vi "Compressor Control.vi"() -> ()   [LabVIEW 2023]
doc: "This VI hosts two shared variables that can be accessed by a variety of client VIs. Shared Variables are typically used for monitoring lossy data, like memory usage, temperature data, etc."
uses:
  CM_Virtual_Panel_LV9_0.llb/Com_Set_AX.ctl
  <vilib>/Instr/_visa.llb/VISA Configure Serial Port (Serial Instr).vi
  <vilib>/Instr/_visa.llb/VISA Configure Serial Port (Instr).vi
panel:
  out "BPP Speed":dbl
  out "BPP status":bool
  out "SPP Speed":dbl
  out "SPP status":bool
  out "String 2":string="Hz"
  out "String":string="Hz"
  out "Unit 2":string="Torr"
  out "BPP Pressure":dbl=0.006515415732577395 format="%#_2e"
  out "Unit 4":string="Torr"
  out "overpressure indicator":bool
  out "Overpressure":bool
  out "Overpressure":bool
  out "output 1":dbl
  out "power":dbl(graph)
  out "Heater Power":string
  out "Cold head pressure":string
  out "Inlet pressure":dbl=1.198
  out "Monitor 1":cluster{"pressure":dbl, "Inlet pressure":dbl}(graph)
  in  "Reading 1":string(combo)="255:R:MRMD"
  out "Unit":string
  out "Unit":string="°C"
  out "Cold Head Temp":dbl=24.81
  out "Motor Current (A)":dbl(knob) scale=0.0..50.0
  out "Compressor Status":bool
  out "Overide status":bool
  out "Comp ON":bool
  out "?":cluster{dbl, dbl, dbl}(slide) scale=32.0..120.0
  out "?":cluster{dbl, dbl, dbl}(slide) scale=32.0..220.0
  out "?":cluster{dbl, dbl, dbl}(slide) scale=32.0..125.0
  out "?":cluster{dbl, dbl, dbl}(slide) scale=32.0..85.0
  out "DP":dbl(knob) scale=0.0..265.0
  in  "CM Tab Control":T1(tab)
  in  "COM PORT SETUP":T2={"Com Port #"=2, "Timeout(ms)"=500, "Baud"=115200, "Slave Address"=16, "LinkMode"=enum."SMDP-II:Checksum and stamp", "Num Retries"=0} {"Slave Address" min=16; "Com Port #" min=1}
  in  "Data Read Length":u32=20
  in  "Pressure Monitor Port":refnum<visa-resource-name>="COM5"
  in  "Command read length":u32=20
  in  "Separation length":i32=10
  in  "Do logging?":bool=TRUE
  in  "Log File Path":path
  out "error out":errorcluster
  out "data feedback":string
  out "command feedback":string
  in  "SPP Off/On":bool
  in  "SPP Standby/Full":bool
  in  "SPP port":refnum<visa-resource-name>
  in  "BPP Off/On":bool
  in  "BPP Standby/Full":bool
  in  "BPP port":refnum<visa-resource-name>
  in  "Set SPP standby speed":dbl=20.0 min=20.0 max=30.0 step=0.3000030517578125 format="%#.1f"
  in  "Set standby speed 3":bool
  out "SPP % full speed":i8 format="%.0f%%"
  in  "Set BPP standby speed":dbl=20.0 min=20.0 max=30.0 step=0.3000030517578125 format="%#.1f"
  out "BPP % full speed":i8 format="%.0f%%"
  out "SPP data out":bool
  out "BPP data out":bool
  in  "Set standby speed4":bool
  out "Gauge":cluster{dbl, dbl, dbl, dbl, dbl, dbl}(knob)={0.0, 0.0, -0.1, 0.0, 0.0, 0.0} scale=0.0..400.0
  in  "Additel 681 Tab Control":enum32{"Gauge Control", "Status"}(tab)
  in  "Zero Reading":bool
  in  "Cancel Zero reading":bool
  out "Gauge battery Voltage":dbl
  in  "Read":bool
  in  "Enable light control":bool
  in  "Gauge light":bool
  in  "Abort monitoring":bool
  out "Battery status":bool
  out "yellow":bool
  out "orange":bool
  out "red":bool
  in  "voltage read length":u32=25
  out "Voltage feedback":string
  in  "monitor 2 read length":u32=25
  out "monitor 2 feedback":string
  in  "monitor 1 read length":u32=25
  out "Monitor 1 feedback":string
  out "Unit":string="°C"
  out "Vapor Temp":dbl=24.81
  out "Monitor 2":dbl(graph)=24.81
  in  "Reading 2":string(combo)="255:R:OTEMP"
  out "Monitor 3":dbl(graph)=0.006479277826451128
  out "SPP Pressure":dbl=0.006479277826451128 format="%#_2e"
  out "Monitor 4":T3(graph)
  in  "Compressor Relay Control":enum32{"Normal", "Overide"}(tab)
  in  "Pressure Upper Limit":dbl=3.0
  out "Helium Overpressure":bool
  in  "Pressure Lower Limit":dbl=1.0
  in  "Set Relay voltage":dbl(slide)=9.0 scale=0.0..10.0
  out "Numeric 2":dbl=9.0
  out "Helium underpressure":bool
  in  "Compressor On":bool caption="Compressor Ona"
  # "Additel Pressure Gauge"
  # "Cryomech Liquefier"
  # "Pressure (Psi)"
  # "Cryomech Control"
  # "Min"
  # "Max"
  # "Latest"
  # "Coolant Supply"
  # "Coolant Return"
  # "Exchage Helium"
  # "Motor Oil"
  # "Temperature °F"
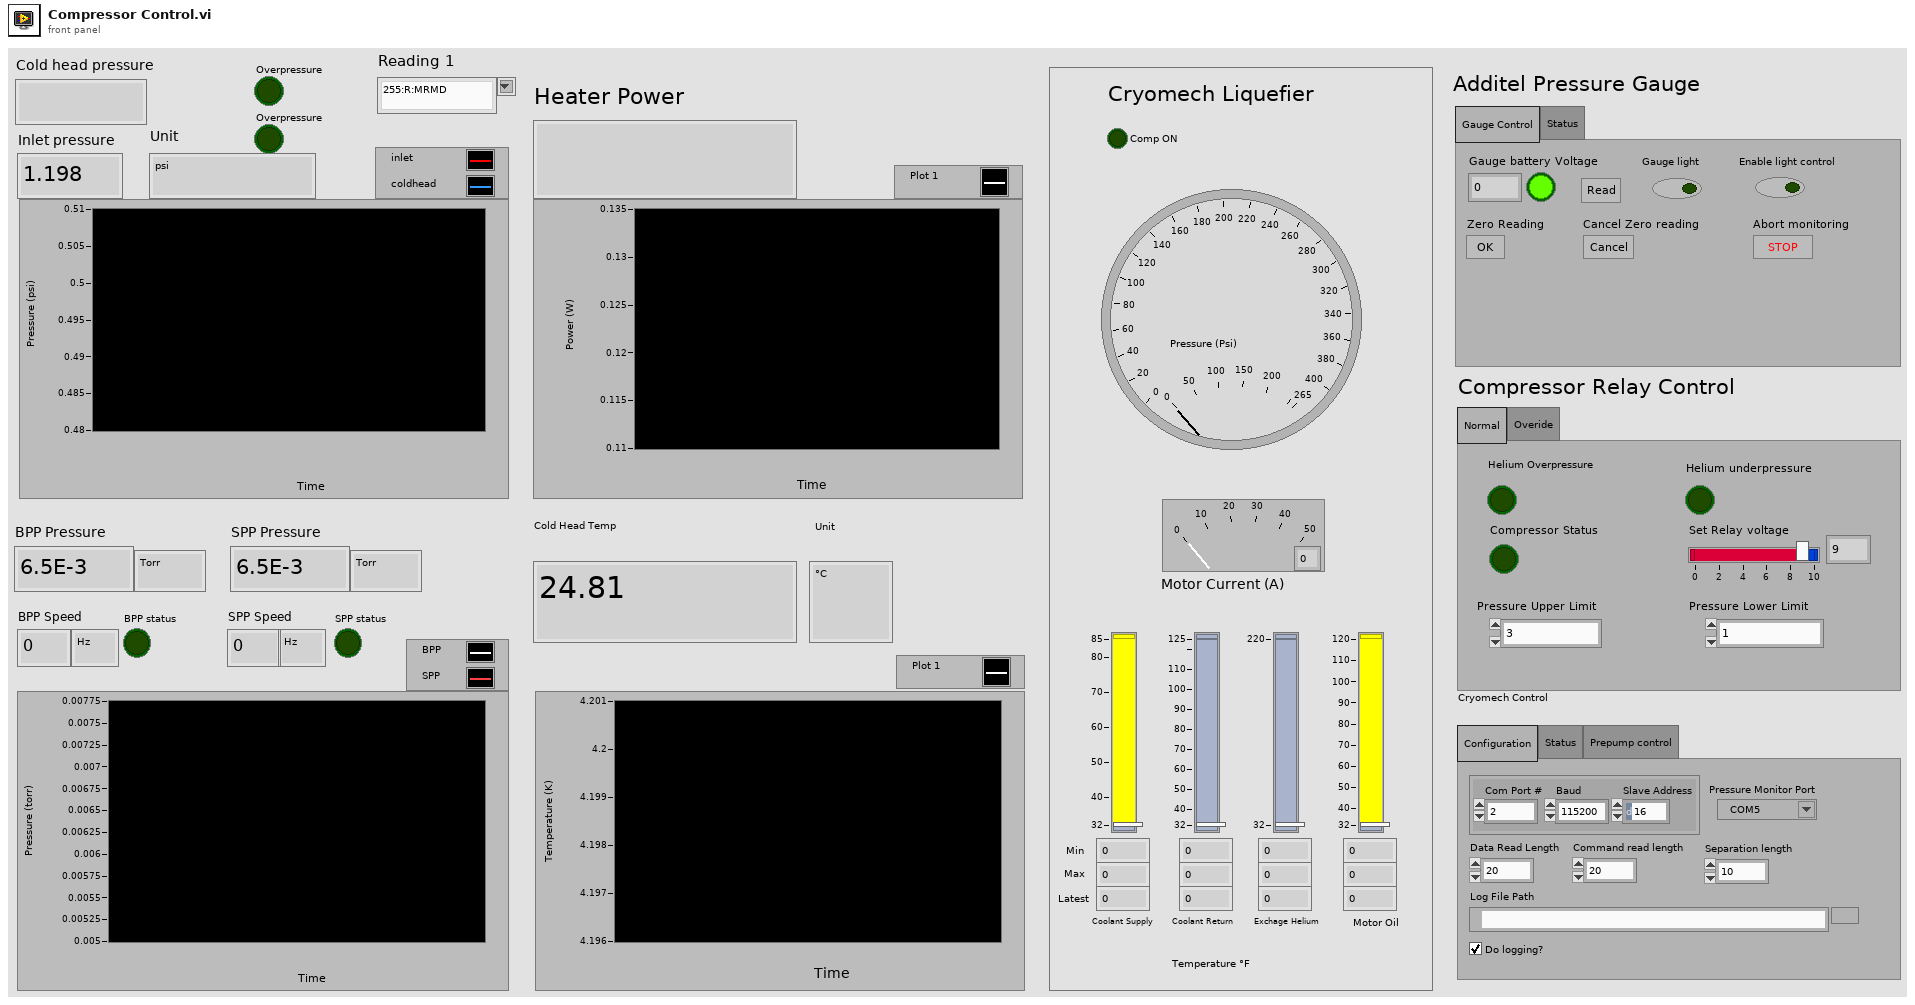
[diagram p1: front panel]
types:
  T1 = enum32{"Configuration", "Status", "Prepump control"}
  T2 = typedef "Com_Set_AX.ctl" = cluster{"Com Port #":u8, "Timeout(ms)":u32, "Baud":u32, "Slave Address":u8, "LinkMode":enum16{"SMDP-I:Checksum, no stamp", "SMDP-II:Checksum and stamp", "Sycon Protocol"}, "Num Retries":u8}
  T3 = cluster{"Output Variable 1":dbl, "Output Variable 2":dbl}
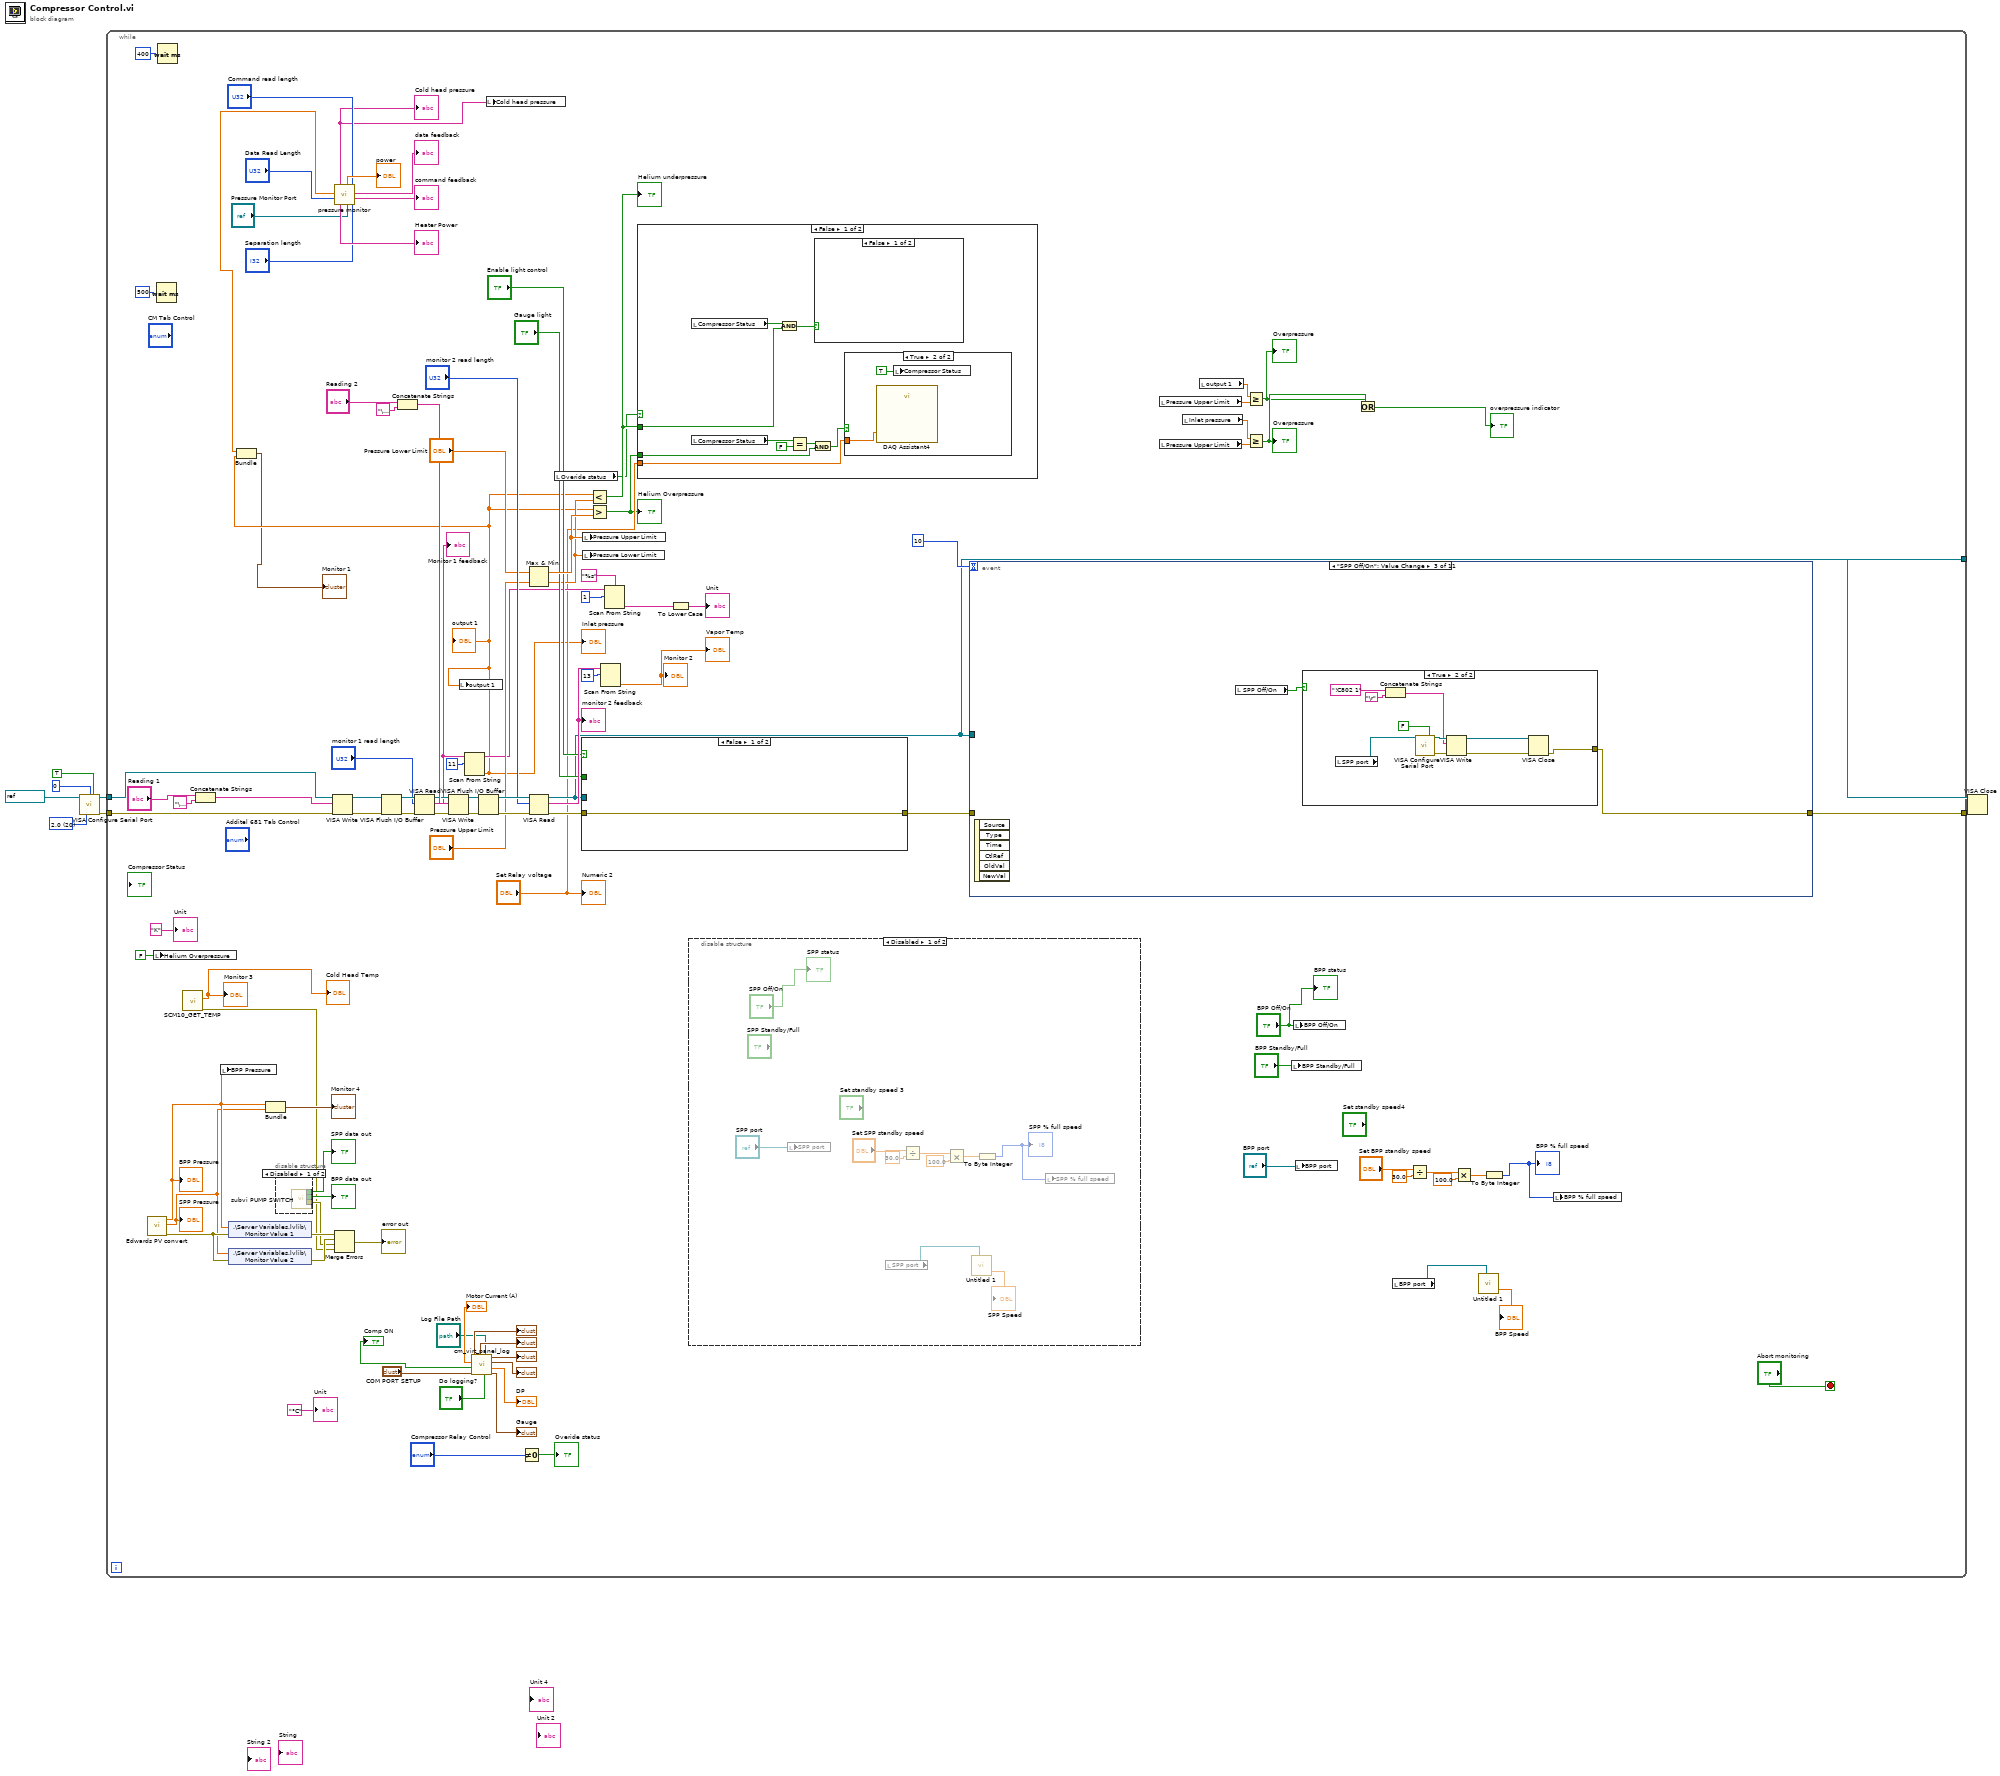
[diagram p0: block diagram]
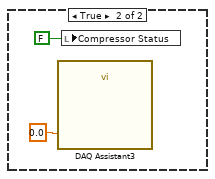
[diagram p4: hidden frame]
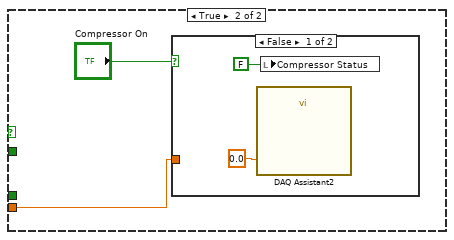
[diagram p6: hidden frame]
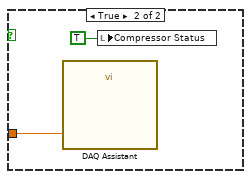
[diagram p7: hidden frame]
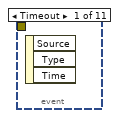
[diagram p8: hidden frame]
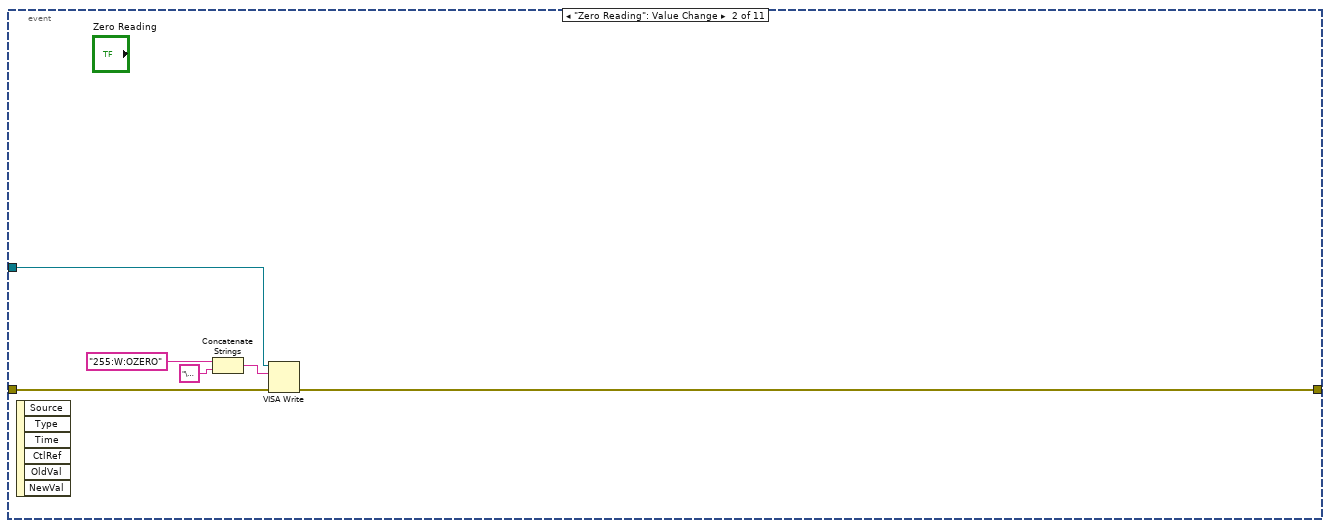
[diagram p9: hidden frame]
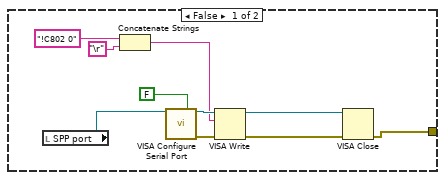
[diagram p10: hidden frame]
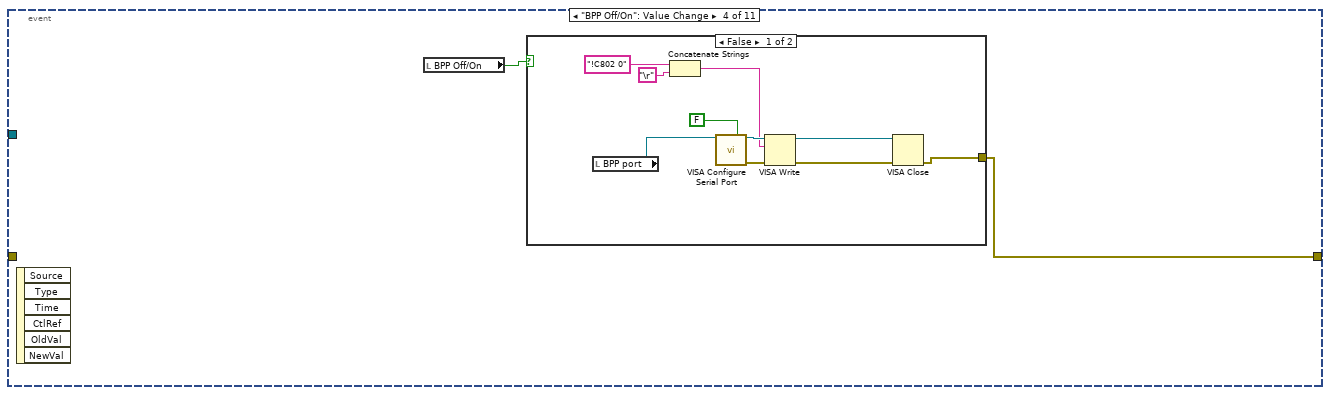
[diagram p11: hidden frame]
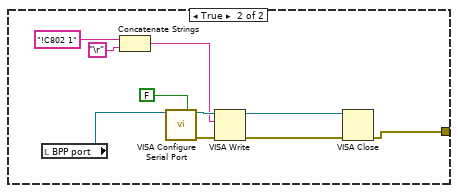
[diagram p12: hidden frame]
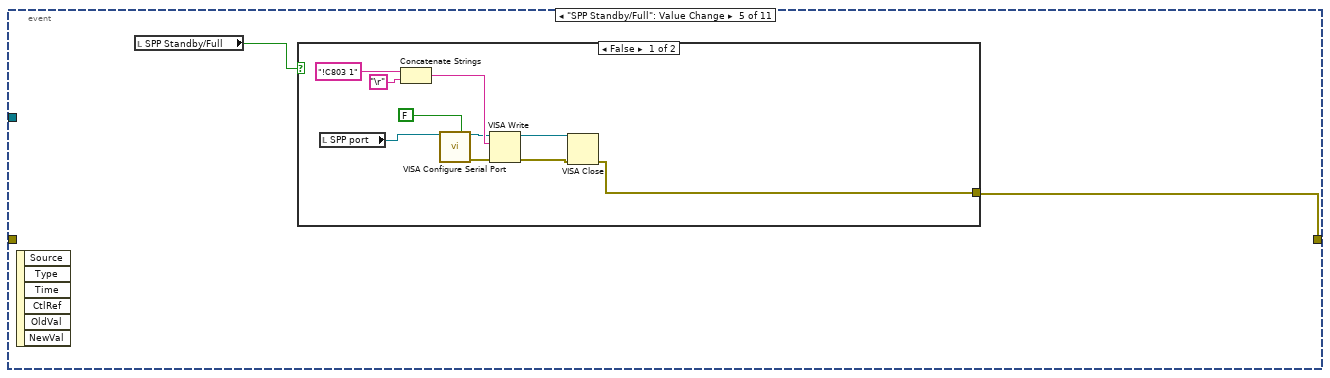
[diagram p13: hidden frame]
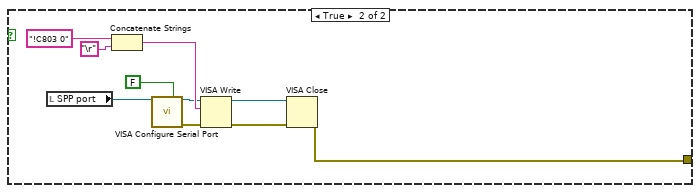
[diagram p14: hidden frame]
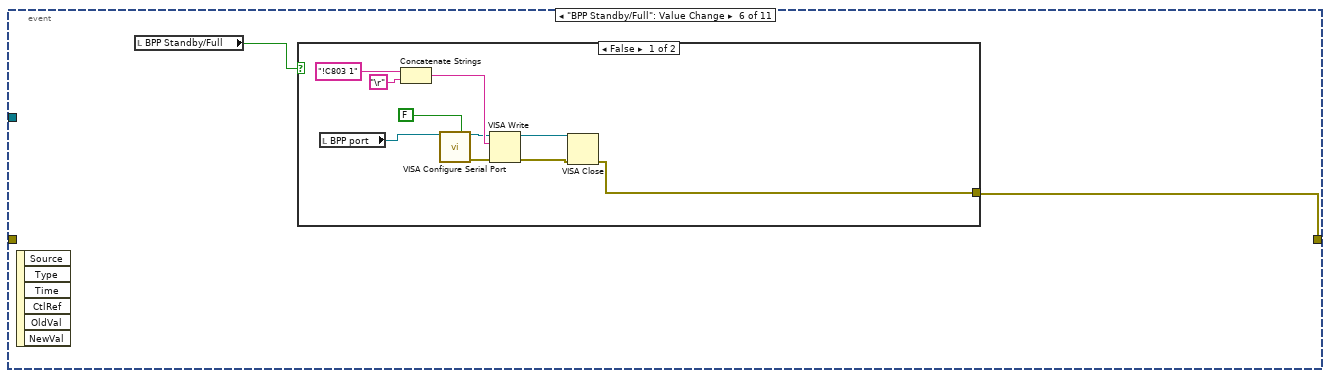
[diagram p15: hidden frame]
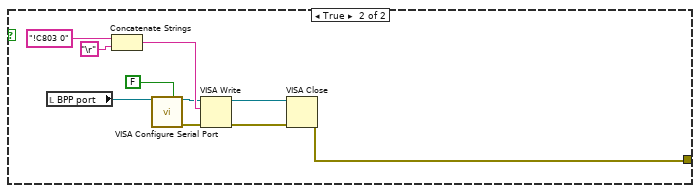
[diagram p16: hidden frame]
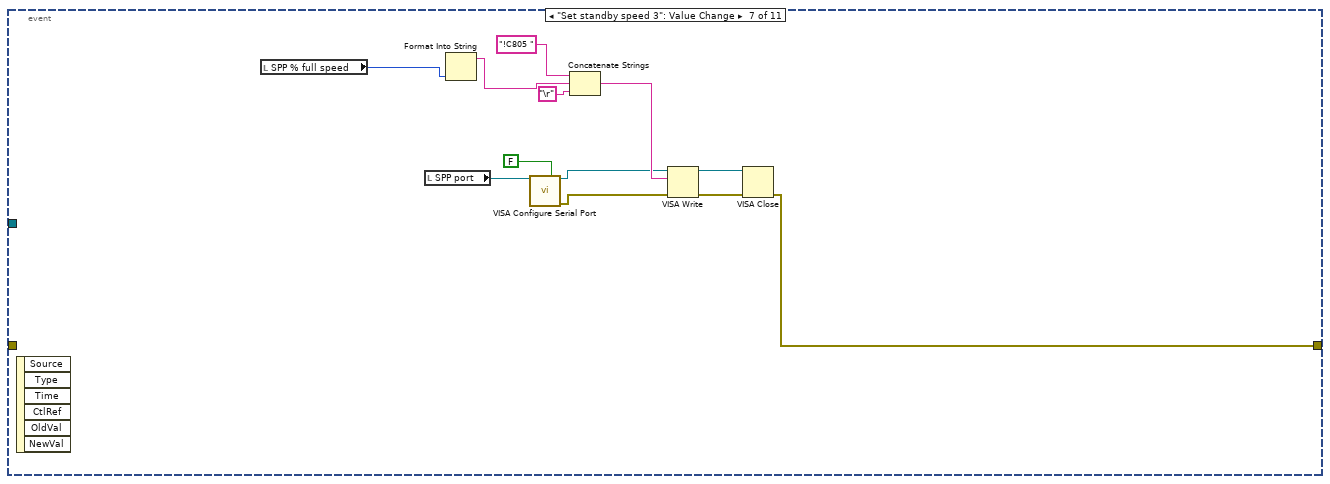
[diagram p17: hidden frame]
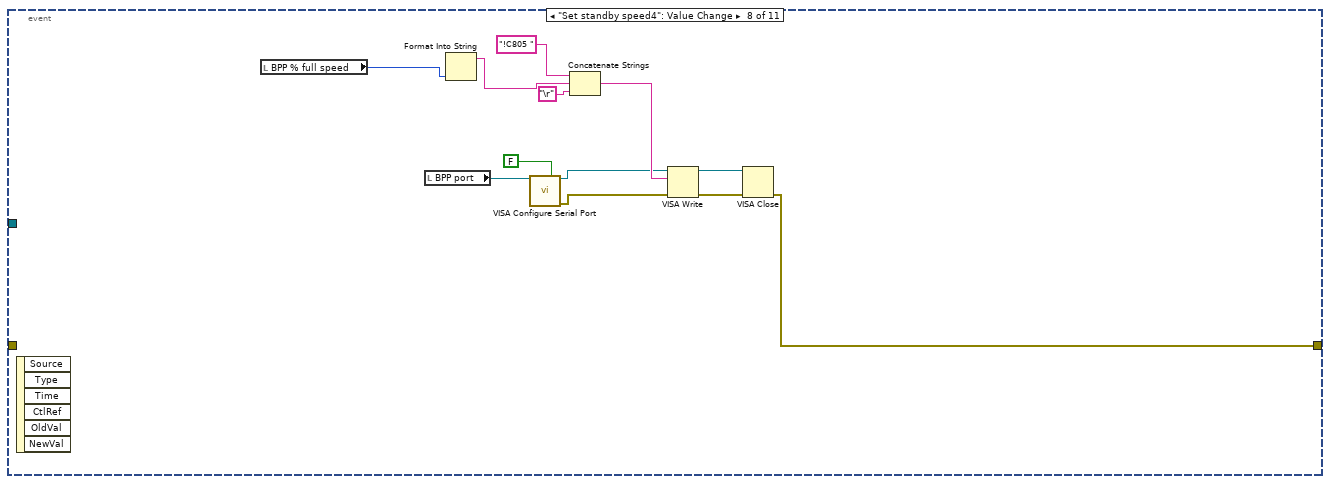
[diagram p18: hidden frame]
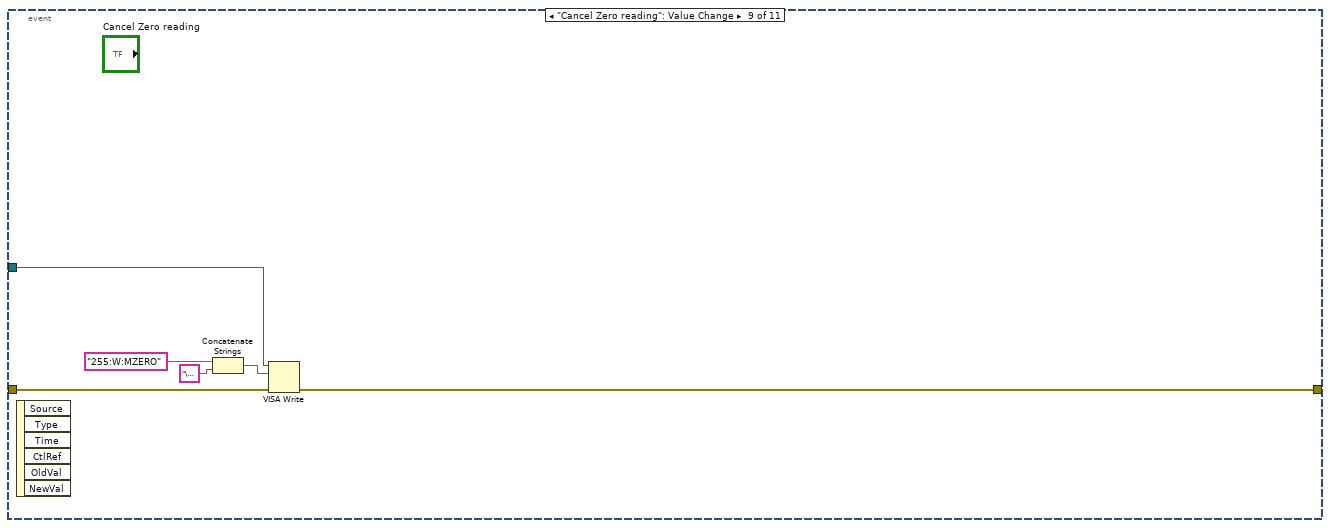
[diagram p19: hidden frame]
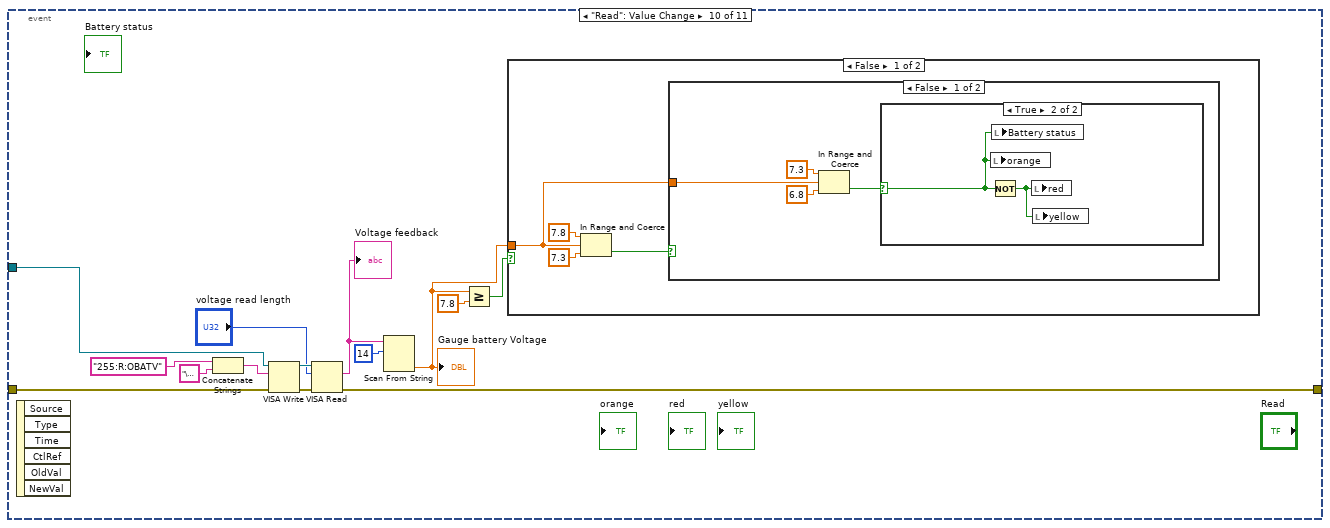
[diagram p20: hidden frame]
diagram:
  w5 = u16 20 items=["1.0"=10, "1.5"=15, "2.0"=20] ("stop bits (10: 1 bit)")
  n1 = call-poly "VISA Configure Serial Port"("VISA resource name"=refnum<visa-resource-name> "COM3", "termination char\n(0xA = '\\n' = LF)"=u8 0 ("termination char\n(0xA = '\\n' = LF)"), "Enable Termination\nChar (T)"=TRUE ("Enable Termination\nChar (T)"), "stop bits (10: 1 bit)"=w5) -> ("VISA resource name out"=w3:refnum<visa-resource-name>, "error out"=w4:errorcluster)  [unwired: 10 in]
  n2 = while {
    tunnel: [w82] -> w2
    tunnel: w4 -> [w61]
    tunnel: w3 -> [w88]
    tunnel: [w81] -> w1
    stop <- "Abort monitoring" stop-if-true
    n3 = call "Edwards PV convert.vi"() -> ("error out"=w64:errorcluster, "Output Variable 2"=w54:dbl, "Output Variable 1"=w55:dbl)  [unwired: 9 in]
    "SPP Pressure" <- w54
    "BPP Pressure" <- w55
    n4 = local write "Helium Overpressure"(FALSE ("Helium Overpressure")) -> ()
    n5 = Wait (ms)(milliseconds to wait=u32 500) -> ()  [unwired: 1 out]
    n6 = Wait (ms)(milliseconds to wait=u32 400) -> ()  [unwired: 1 out]
    n7 = call "SCM10_GET_TEMP.vi"() -> ("ERR OUT"=w52:errorcluster, "Temperature (K)"=→"Monitor 3" →"Cold Head Temp":dbl)  [unwired: 9 in, 1 out]
    n8 = Concatenate Strings("Reading 1", "\u0000") -> (w114:string)
    n9 = local write "BPP Pressure"(w55) -> ()
    n10 = shared-variable ".\\Server Variables.lvlib\\Monitor Value 1"(w55, error in=w64) -> (error out=w63:errorcluster)
    n11 = shared-variable ".\\Server Variables.lvlib\\Monitor Value 2"(w54, error in=w64) -> (error out=w62:errorcluster)
    n12 = Bundle("Output Variable 1"=w55, "Output Variable 2"=w54) -> (→"Monitor 4":T3)  [unwired: 1 in]
    n13 = disable-structure shown="Disabled" {
      disable-tunnel: [w117 _] -> w69
      disable-tunnel: [w116 _] -> w68
      disable-tunnel: [w115 _] -> w60
      frame Disabled {
        n14 = call "subvi PUMP SWITCH.vi"() -> ("error out"=w115:errorcluster, "data out"=w117:bool, "data out 2"=w116:bool)  [unwired: 9 in]
      }
      frame Enabled {
      }
    }
    "BPP data out" <- w69
    "SPP data out" <- w68
    n15 = VISA Write(VISA resource name=w88, write buffer=w114, error in (no error)=w61) -> (VISA resource name out=w110:refnum<visa-resource-name>, error out=w112:errorcluster)  [unwired: 1 out]
    n16 = call "pressure monitor.vi"("Data Read Length"="Data Read Length", "Pressure Monitor Port"="Pressure Monitor Port", "Command read length"="Command read length", "Separation length"="Separation length") -> ("Cold head pressure"=w24:string, "pressure"=w23:dbl, "Heater Power"=→"Heater Power":string, "power"=→"power":dbl, "data feedback"=→"data feedback":string, "command feedback"=→"command feedback":string)
    "Cold head pressure" <- w24
    n17 = Merge Errors(w63, w62, w60, w52) -> (→"error out":errorcluster)
    n18 = VISA Flush I/O Buffer(VISA resource name=w110, error in (no error)=w112) -> (VISA resource name out=w111:refnum<visa-resource-name>, error out=w107:errorcluster)  [unwired: 1 in]
    n19 = Concatenate Strings("Reading 2", "\u0000") -> (w103:string)
    n20 = VISA Read(VISA resource name=w111, byte count="monitor 1 read length", error in (no error)=w107) -> (VISA resource name out=w93:refnum<visa-resource-name>, read buffer=w79:string, error out=w92:errorcluster)  [unwired: 1 out]
    "Monitor 1 feedback" <- w79
    n21 = VISA Write(VISA resource name=w93, write buffer=w103, error in (no error)=w92) -> (VISA resource name out=w99:refnum<visa-resource-name>, error out=w101:errorcluster)  [unwired: 1 out]
    n22 = Scan From String(input string=w79, initial scan location=u32 11) -> (remaining string=w77:string, output 1=w22:dbl)  [unwired: 3 in, 2 out]
    "Inlet pressure" <- w22
    "output 1" <- w22
    n23 = Bundle("pressure"=w23, "Inlet pressure"=w22) -> (→"Monitor 1":cluster{"pressure":dbl, "Inlet pressure":dbl})  [unwired: 1 in]
    n24 = local write "output 1"(w22) -> ()
    n25 = call "cm_virt_panel_log.vi"("Do logging?"="Do logging?", "Log File Path"="Log File Path", "COM PORT SETUP"="COM PORT SETUP") -> ("Gauge"=→"Gauge":cluster{dbl, dbl, dbl, dbl, dbl, dbl}, "DP"=→"DP":dbl, "H2O IN"=→"?":cluster{dbl, dbl, dbl}, "H2O OUT"=→"?":cluster{dbl, dbl, dbl}, "He GAS"=→"?":cluster{dbl, dbl, dbl}, "Comp ON"=→"Comp ON":bool, "Motor Amps"=→"Motor Current (A)":dbl, "OIL TEMP"=→"?":cluster{dbl, dbl, dbl})  [unwired: 1 in]
    n26 = VISA Flush I/O Buffer(VISA resource name=w99, error in (no error)=w101) -> (VISA resource name out=w100:refnum<visa-resource-name>, error out=w95:errorcluster)  [unwired: 1 in]
    n27 = local write "Cold head pressure"(w24) -> ()
    n28 = Not Equal To 0?(x="Compressor Relay Control") -> (x != 0?=→"Overide status":bool)
    n29 = Max & Min(x="Pressure Lower Limit", y="Pressure Upper Limit") -> (max(x,y)=w89:dbl, min(x,y)=w73:dbl)
    n30 = VISA Read(VISA resource name=w100, byte count="monitor 2 read length", error in (no error)=w95) -> (VISA resource name out=w82:refnum<visa-resource-name>, read buffer=w97:string, error out=w85:errorcluster)  [unwired: 1 out]
    "monitor 2 feedback" <- w97
    n31 = local read "Overide status"() -> (w58:bool)
    n32 = case shown="False" "Enable light control" {
      tunnel: "Gauge light" -> [_ w319]
      tunnel: w85 -> [w315 w318]
      tunnel: [w315 w317] -> w80
      tunnel: w82 -> [_ w316]
      frame False {
      }
      frame True {
        n33 = case shown="False" w319 {
          tunnel: w316 -> [w322 w331]
          tunnel: [w321 w327] -> w317
          tunnel: w318 -> [w320 w326]
          frame False {
            n34 = Concatenate Strings("255:W:OBLAC:0" ("string"), "\u0000" ("string")) -> (w323:string)
            n35 = VISA Write(VISA resource name=w322, write buffer=w323, error in (no error)=w320) -> (error out=w321:errorcluster)  [unwired: 2 out]
          }
          frame True {
            n36 = Concatenate Strings("255:W:OBLAC:1" ("string"), "\u0000" ("string")) -> (w328:string)
            n37 = VISA Write(VISA resource name=w331, write buffer=w328, error in (no error)=w326) -> (error out=w327:errorcluster)  [unwired: 2 out]
          }
        }
      }
    }
    n38 = local write "Pressure Upper Limit"(w89) -> ()
    n39 = local write "Pressure Lower Limit"(w73) -> ()
    n40 = Less?(x=w22, y=w73) -> (x < y?=w65:bool)
    "Helium underpressure" <- w65
    n41 = Greater?(x=w22, y=w89) -> (0:w66:bool)
    "Helium Overpressure" <- w66
    n42 = Scan From String(input string=w97, initial scan location=u32 13) -> (output 1=→"Vapor Temp" →"Monitor 2":dbl)  [unwired: 3 in, 3 out]
    n43 = Scan From String(format string="%s", input string=w77, initial scan location=u32 1) -> (output 1=w75:string)  [unwired: 2 in, 3 out]
    n44 = case shown="False" w58 {
      tunnel: "Set Relay voltage" -> [w133 w141]
      tunnel: w66 -> [w129 _]
      tunnel: w65 -> [w128 _]
      frame False {
        n45 = local read "Compressor Status"() -> (w136:bool)
        n46 = local read "Compressor Status"() -> (w132:bool)
        n47 = And(x=w136, y=w128) -> (x .and. y?=w135:bool)
        n48 = Equal?(x=w132, y=FALSE) -> (x = y?=w130:bool)
        n49 = And(x=w130, y=w129) -> (x .and. y?=w134:bool)
        n50 = case shown="False" w135 {
          frame False {
          }
          frame True {
            n51 = call "DAQ Assistant3"("data"=0.0) -> ()  [unwired: 17 in, 2 out]
            n52 = local write "Compressor Status"(FALSE ("Compressor Status")) -> ()
          }
        }
        n53 = case shown="True" w134 {
          tunnel: w133 -> [_ w140]
          frame False {
          }
          frame True {
            n54 = call "DAQ Assistant4"("data"=w140) -> ()  [unwired: 17 in, 2 out]
            n55 = local write "Compressor Status"(TRUE ("Compressor Status")) -> ()
          }
        }
      }
      frame True {
        n56 = case shown="False" "Compressor On" {
          tunnel: w141 -> [_ w146]
          frame False {
            n57 = call "DAQ Assistant2"("data"=0.0) -> ()  [unwired: 17 in, 2 out]
            n58 = local write "Compressor Status"(FALSE ("Compressor Status")) -> ()
          }
          frame True {
            n59 = call "DAQ Assistant"("data"=w146) -> ()  [unwired: 17 in, 2 out]
            n60 = local write "Compressor Status"(TRUE ("Compressor Status")) -> ()
          }
        }
      }
    }
    n61 = To Lower Case(string=w75) -> (all lower case string=→"Unit":string)
    n62 = disable-structure shown="Disabled" {
      frame Disabled {
        n63 = local write "SPP port"("SPP port") -> ()
        n64 = local read "SPP port"() -> (w118:refnum<visa-resource-name>)
        n65 = Divide(x="Set SPP standby speed", y=30.0) -> (x/y=w124:dbl)
        n66 = Multiply(x=w124, y=sgl 100.0) -> (x*y=w127:dbl)
        n67 = call "Untitled 1.vi"("VISA resource name"=w118) -> ("Speed"=→"SPP Speed":dbl)  [unwired: 10 in]
        n68 = To Byte Integer(number=w127) -> (8bit integer=w120:i8)
        "SPP % full speed" <- w120
        n69 = local write "SPP % full speed"(w120) -> ()
        "SPP status" <- "SPP Off/On"
      }
      frame Enabled {
      }
    }
    n70 = event shown="[2] \"SPP Off/On\": Value Change" {
      selector: _ -> [_ _ _ _ _ _ _ _ _ _ _]
      dyn-events: _ -> [_ _ _ _ _ _ _ _ _ _ _]
      timeout: 10 -> [_ _ _ _ _ _ _ _ _ _ _]
      tunnel: w82 -> [_ w147 _ _ _ _ _ _ w266 w276 _]
      tunnel: [_ w148 w153 w175 w197 w219 w241 w253 w265 w275 _] -> w81
      tunnel: w80 -> [_ w149 _ _ _ _ _ _ w267 w272 _]
      event Timeout {
        n71 = event-data() -> ()  [unwired: 1 in, 3 out]
      }
      event "Zero Reading": Value Change {
        n72 = event-data() -> ()  [unwired: 1 in, 6 out]
        n73 = Concatenate Strings("255:W:OZERO" ("string"), "\u0000" ("string")) -> (w150:string)
        n74 = VISA Write(VISA resource name=w147, write buffer=w150, error in (no error)=w149) -> (error out=w148:errorcluster)  [unwired: 2 out]
      }
      event "SPP Off/On": Value Change {
        n75 = event-data() -> ()  [unwired: 1 in, 6 out]
        n76 = local read "SPP Off/On"() -> (w154:bool)
        n77 = case shown="True" w154 {
          tunnel: [w158 w168] -> w153
          frame False {
            n78 = local read "SPP port"() -> (w157:refnum<visa-resource-name>)
            n79 = Concatenate Strings("!C802 0" ("string"), "\r" ("string")) -> (w159:string)
            n80 = call-poly "VISA Configure Serial Port"("VISA resource name"=w157, "Enable Termination\nChar (T)"=FALSE ("Enable Termination\nChar (T)")) -> ("VISA resource name out"=w164:refnum<visa-resource-name>, "error out"=w163:errorcluster)  [unwired: 12 in]
            n81 = VISA Write(VISA resource name=w164, write buffer=w159, error in (no error)=w163) -> (VISA resource name out=w156:refnum<visa-resource-name>, error out=w155:errorcluster)  [unwired: 1 out]
            n82 = VISA Close(VISA resource name=w156, error in (no error)=w155) -> (error out=w158:errorcluster)
          }
          frame True {
            n83 = local read "SPP port"() -> (w167:refnum<visa-resource-name>)
            n84 = Concatenate Strings("!C802 1" ("string"), "\r" ("string")) -> (w169:string)
            n85 = call-poly "VISA Configure Serial Port"("VISA resource name"=w167, "Enable Termination\nChar (T)"=FALSE ("Enable Termination\nChar (T)")) -> ("VISA resource name out"=w174:refnum<visa-resource-name>, "error out"=w173:errorcluster)  [unwired: 12 in]
            n86 = VISA Write(VISA resource name=w174, write buffer=w169, error in (no error)=w173) -> (VISA resource name out=w166:refnum<visa-resource-name>, error out=w165:errorcluster)  [unwired: 1 out]
            n87 = VISA Close(VISA resource name=w166, error in (no error)=w165) -> (error out=w168:errorcluster)
          }
        }
      }
      event "BPP Off/On": Value Change {
        n88 = event-data() -> ()  [unwired: 1 in, 6 out]
        n89 = local read "BPP Off/On"() -> (w176:bool)
        n90 = case shown="False" w176 {
          tunnel: [w180 w190] -> w175
          frame False {
            n91 = local read "BPP port"() -> (w179:refnum<visa-resource-name>)
            n92 = Concatenate Strings("!C802 0" ("string"), "\r" ("string")) -> (w181:string)
            n93 = call-poly "VISA Configure Serial Port"("VISA resource name"=w179, "Enable Termination\nChar (T)"=FALSE ("Enable Termination\nChar (T)")) -> ("VISA resource name out"=w186:refnum<visa-resource-name>, "error out"=w185:errorcluster)  [unwired: 12 in]
            n94 = VISA Write(VISA resource name=w186, write buffer=w181, error in (no error)=w185) -> (VISA resource name out=w178:refnum<visa-resource-name>, error out=w177:errorcluster)  [unwired: 1 out]
            n95 = VISA Close(VISA resource name=w178, error in (no error)=w177) -> (error out=w180:errorcluster)
          }
          frame True {
            n96 = local read "BPP port"() -> (w189:refnum<visa-resource-name>)
            n97 = Concatenate Strings("!C802 1" ("string"), "\r" ("string")) -> (w191:string)
            n98 = call-poly "VISA Configure Serial Port"("VISA resource name"=w189, "Enable Termination\nChar (T)"=FALSE ("Enable Termination\nChar (T)")) -> ("VISA resource name out"=w196:refnum<visa-resource-name>, "error out"=w195:errorcluster)  [unwired: 12 in]
            n99 = VISA Write(VISA resource name=w196, write buffer=w191, error in (no error)=w195) -> (VISA resource name out=w188:refnum<visa-resource-name>, error out=w187:errorcluster)  [unwired: 1 out]
            n100 = VISA Close(VISA resource name=w188, error in (no error)=w187) -> (error out=w190:errorcluster)
          }
        }
      }
      event "SPP Standby/Full": Value Change {
        n101 = event-data() -> ()  [unwired: 1 in, 6 out]
        n102 = local read "SPP Standby/Full"() -> (w198:bool)
        n103 = case shown="False" w198 {
          tunnel: [w199 w209] -> w197
          frame False {
            n104 = local read "SPP port"() -> (w204:refnum<visa-resource-name>)
            n105 = Concatenate Strings("!C803 1" ("string"), "\r") -> (w208:string)
            n106 = call-poly "VISA Configure Serial Port"("VISA resource name"=w204, "Enable Termination\nChar (T)"=FALSE ("Enable Termination\nChar (T)")) -> ("VISA resource name out"=w203:refnum<visa-resource-name>, "error out"=w202:errorcluster)  [unwired: 12 in]
            n107 = VISA Write(VISA resource name=w203, write buffer=w208, error in (no error)=w202) -> (VISA resource name out=w201:refnum<visa-resource-name>, error out=w200:errorcluster)  [unwired: 1 out]
            n108 = VISA Close(VISA resource name=w201, error in (no error)=w200) -> (error out=w199:errorcluster)
          }
          frame True {
            n109 = local read "SPP port"() -> (w215:refnum<visa-resource-name>)
            n110 = Concatenate Strings("!C803 0" ("string"), "\r") -> (w218:string)
            n111 = call-poly "VISA Configure Serial Port"("VISA resource name"=w215, "Enable Termination\nChar (T)"=FALSE ("Enable Termination\nChar (T)")) -> ("VISA resource name out"=w213:refnum<visa-resource-name>, "error out"=w212:errorcluster)  [unwired: 12 in]
            n112 = VISA Write(VISA resource name=w213, write buffer=w218, error in (no error)=w212) -> (VISA resource name out=w211:refnum<visa-resource-name>, error out=w210:errorcluster)  [unwired: 1 out]
            n113 = VISA Close(VISA resource name=w211, error in (no error)=w210) -> (error out=w209:errorcluster)
          }
        }
      }
      event "BPP Standby/Full": Value Change {
        n114 = event-data() -> ()  [unwired: 1 in, 6 out]
        n115 = local read "BPP Standby/Full"() -> (w220:bool)
        n116 = case shown="False" w220 {
          tunnel: [w221 w231] -> w219
          frame False {
            n117 = local read "BPP port"() -> (w226:refnum<visa-resource-name>)
            n118 = Concatenate Strings("!C803 1" ("string"), "\r") -> (w230:string)
            n119 = call-poly "VISA Configure Serial Port"("VISA resource name"=w226, "Enable Termination\nChar (T)"=FALSE ("Enable Termination\nChar (T)")) -> ("VISA resource name out"=w225:refnum<visa-resource-name>, "error out"=w224:errorcluster)  [unwired: 12 in]
            n120 = VISA Write(VISA resource name=w225, write buffer=w230, error in (no error)=w224) -> (VISA resource name out=w223:refnum<visa-resource-name>, error out=w222:errorcluster)  [unwired: 1 out]
            n121 = VISA Close(VISA resource name=w223, error in (no error)=w222) -> (error out=w221:errorcluster)
          }
          frame True {
            n122 = local read "BPP port"() -> (w237:refnum<visa-resource-name>)
            n123 = Concatenate Strings("!C803 0" ("string"), "\r") -> (w240:string)
            n124 = call-poly "VISA Configure Serial Port"("VISA resource name"=w237, "Enable Termination\nChar (T)"=FALSE ("Enable Termination\nChar (T)")) -> ("VISA resource name out"=w235:refnum<visa-resource-name>, "error out"=w234:errorcluster)  [unwired: 12 in]
            n125 = VISA Write(VISA resource name=w235, write buffer=w240, error in (no error)=w234) -> (VISA resource name out=w233:refnum<visa-resource-name>, error out=w232:errorcluster)  [unwired: 1 out]
            n126 = VISA Close(VISA resource name=w233, error in (no error)=w232) -> (error out=w231:errorcluster)
          }
        }
      }
      event "Set standby speed 3": Value Change {
        n127 = event-data() -> ()  [unwired: 1 in, 6 out]
        n128 = local read "SPP % full speed"() -> (w248:i8)
        n129 = local read "SPP port"() -> (w246:refnum<visa-resource-name>)
        n130 = Format Into String(w248) -> (resulting string=w250:string)  [unwired: 3 in, 1 out]
        n131 = call-poly "VISA Configure Serial Port"("VISA resource name"=w246, "Enable Termination\nChar (T)"=FALSE ("Enable Termination\nChar (T)")) -> ("VISA resource name out"=w245:refnum<visa-resource-name>, "error out"=w244:errorcluster)  [unwired: 12 in]
        n132 = Concatenate Strings("!C805 " ("string"), w250, "\r" ("string")) -> (w252:string)
        n133 = VISA Write(VISA resource name=w245, write buffer=w252, error in (no error)=w244) -> (VISA resource name out=w243:refnum<visa-resource-name>, error out=w242:errorcluster)  [unwired: 1 out]
        n134 = VISA Close(VISA resource name=w243, error in (no error)=w242) -> (error out=w241:errorcluster)
      }
      event "Set standby speed4": Value Change {
        n135 = event-data() -> ()  [unwired: 1 in, 6 out]
        n136 = local read "BPP % full speed"() -> (w260:i8)
        n137 = local read "BPP port"() -> (w258:refnum<visa-resource-name>)
        n138 = Format Into String(w260) -> (resulting string=w262:string)  [unwired: 3 in, 1 out]
        n139 = call-poly "VISA Configure Serial Port"("VISA resource name"=w258, "Enable Termination\nChar (T)"=FALSE ("Enable Termination\nChar (T)")) -> ("VISA resource name out"=w257:refnum<visa-resource-name>, "error out"=w256:errorcluster)  [unwired: 12 in]
        n140 = Concatenate Strings("!C805 " ("string"), w262, "\r" ("string")) -> (w264:string)
        n141 = VISA Write(VISA resource name=w257, write buffer=w264, error in (no error)=w256) -> (VISA resource name out=w255:refnum<visa-resource-name>, error out=w254:errorcluster)  [unwired: 1 out]
        n142 = VISA Close(VISA resource name=w255, error in (no error)=w254) -> (error out=w253:errorcluster)
      }
      event "Cancel Zero reading": Value Change {
        n143 = event-data() -> ()  [unwired: 1 in, 6 out]
        n144 = Concatenate Strings("255:W:MZERO" ("string"), "\u0000" ("string")) -> (w270:string)
        n145 = VISA Write(VISA resource name=w266, write buffer=w270, error in (no error)=w267) -> (error out=w265:errorcluster)  [unwired: 2 out]
      }
      event "Read": Value Change {
        n146 = event-data() -> ()  [unwired: 1 in, 6 out]
        n147 = Concatenate Strings("255:R:OBATV" ("string"), "\u0000" ("string")) -> (w282:string)
        n148 = VISA Write(VISA resource name=w276, write buffer=w282, error in (no error)=w272) -> (VISA resource name out=w280:refnum<visa-resource-name>, error out=w281:errorcluster)  [unwired: 1 out]
        n149 = VISA Read(VISA resource name=w280, byte count="voltage read length", error in (no error)=w281) -> (read buffer=w278:string, error out=w275:errorcluster)  [unwired: 2 out]
        "Voltage feedback" <- w278
        n150 = Scan From String(input string=w278, initial scan location=u32 14) -> (output 1=w271:dbl)  [unwired: 3 in, 3 out]
        "Gauge battery Voltage" <- w271
        n151 = Greater Or Equal?(x=w271, y=7.8) -> (x >= y?=w273:bool)
        n152 = case shown="False" w273 {
          selector: w273 -> [_ w300]
          tunnel: w271 -> [w285 _]
          frame False {
            n153 = In Range and Coerce(upper limit=7.8, x=w285, lower limit=7.3) -> (In Range?=w286:bool)  [unwired: 1 out]
            n154 = case shown="False" w286 {
              selector: w286 -> [_ w298]
              tunnel: w285 -> [w292 _]
              frame False {
                n155 = In Range and Coerce(upper limit=7.3, x=w292, lower limit=6.8) -> (In Range?=w289:bool)  [unwired: 1 out]
                n156 = case shown="True" w289 {
                  selector: w289 -> [w294 w296]
                  frame False {
                    n157 = local write "yellow"(w294) -> ()
                    n158 = Not(x=w294) -> (.not. x?=w293:bool)
                    n159 = local write "orange"(w294) -> ()
                    n160 = local write "red"(w293) -> ()
                    n161 = local write "Battery status"(w293) -> ()
                  }
                  frame True {
                    n162 = Not(x=w296) -> (.not. x?=w295:bool)
                    n163 = local write "orange"(w296) -> ()
                    n164 = local write "Battery status"(w296) -> ()
                    n165 = local write "red"(w295) -> ()
                    n166 = local write "yellow"(w295) -> ()
                  }
                }
              }
              frame True {
                n167 = local write "yellow"(w298) -> ()
                n168 = Not(x=w298) -> (.not. x?=w297:bool)
                n169 = local write "Battery status"(w298) -> ()
                n170 = local write "red"(w297) -> ()
                n171 = local write "orange"(w297) -> ()
              }
            }
          }
          frame True {
            n172 = Not(x=w300) -> (.not. x?=w299:bool)
            n173 = local write "red"(w299) -> ()
            n174 = local write "yellow"(w299) -> ()
            n175 = local write "orange"(w299) -> ()
            n176 = local write "Battery status"(w299) -> ()
          }
        }
      }
      event "overpressure indicator": Value Change {
        n177 = event-data() -> ()  [unwired: 1 in, 6 out]
        n178 = local read "Inlet pressure"() -> (w304:dbl)
        n179 = local read "Cold head pressure"() -> (w305:string)
        n180 = Format Into String(w304) -> (resulting string=w303:string)  [unwired: 3 in, 1 out]
        n181 = Get Date/Time String(date format (0)=enum16{"short", "long", "abbreviated"}."abbreviated") -> (date string=w310:string, time string=w311:string)  [unwired: 2 in]
        n182 = Concatenate Strings("Coldhead :", w305, ", inlet:" ("string"), w303, "." ("string")) -> (w313:string)
        n183 = Concatenate Strings("Helium overpressure on ", w310, " " ("string"), w311, ". Helium pressures are: " ("string"), w313) -> (w314:string)
        n184 = call "Send Email"("Message"=w314) -> ()  [unwired: 10 in, 1 out]
      }
    }
    n185 = local read "Pressure Upper Limit"() -> (w46:dbl)
    n186 = local read "Pressure Upper Limit"() -> (w45:dbl)
    n187 = local read "Inlet pressure"() -> (w50:dbl)
    n188 = local read "output 1"() -> (w49:dbl)
    n189 = Greater Or Equal?(x=w49, y=w46) -> (x >= y?=w47:bool)
    "Overpressure" <- w47
    n190 = Greater Or Equal?(x=w50, y=w45) -> (x >= y?=w48:bool)
    "Overpressure" <- w48
    n191 = local write "BPP Standby/Full"("BPP Standby/Full") -> ()
    n192 = local write "BPP Off/On"("BPP Off/On") -> ()
    n193 = local write "BPP port"("BPP port") -> ()
    n194 = Or(x=w48, y=w47) -> (x .or. y?=→"overpressure indicator":bool)
    n195 = local read "BPP port"() -> (w10:refnum<visa-resource-name>)
    n196 = Divide(x="Set BPP standby speed", y=30.0) -> (x/y=w17:dbl)
    n197 = Multiply(x=w17, y=sgl 100.0) -> (x*y=w20:dbl)
    n198 = call "Untitled 1.vi"("VISA resource name"=w10) -> ("Speed"=→"BPP Speed":dbl)  [unwired: 10 in]
    n199 = To Byte Integer(number=w20) -> (8bit integer=w12:i8)
    "BPP % full speed" <- w12
    n200 = local write "BPP % full speed"(w12) -> ()
    "Unit" <- "°C" ("Unit")
    "Numeric 2" <- "Set Relay voltage"
    "Unit" <- "K" ("Unit")
    "BPP status" <- "BPP Off/On"
  }
  n201 = VISA Close(VISA resource name=w2, error in (no error)=w1) -> ()  [unwired: 1 out]
